vi "Swap DDS with CS.vi"(6 "Variant in":variant, 7 "Shift Pressed?":bool, 8 "error in (no error)":errorcluster, 10 "QD Combo Box Ref":refnum<vi>, 11 "QD Launch VI Ref":refnum<vi>) -> (0 "error out":errorcluster, 4 "Variant out":variant)   [LabVIEW 2017]
doc: "PLUGIN_DESCRIPTION: Replaces selected Diagram Disable Structure with Case Structure. Based on SAPHIR_DisableCode.vi from https://forums.ni.com/t5/SAPHIR-Toolkits-Documents/ViBox-Quick-Drop-datasheet/ta-p/3507939?profile.language=en\nPLUGIN_DEFAULT_SHORTCUT:"
uses:
  <userlib>/_LAVACR/Scripting Tools/Scripting Tools.lvlib
panel:
  in  "Undo Name":string="DisableCode"
  # "Created by https://github.com/Zieleslaw/, based on:"
  # "More informations on : https://decibel.ni.com/content/groups/saphir-toolkit"
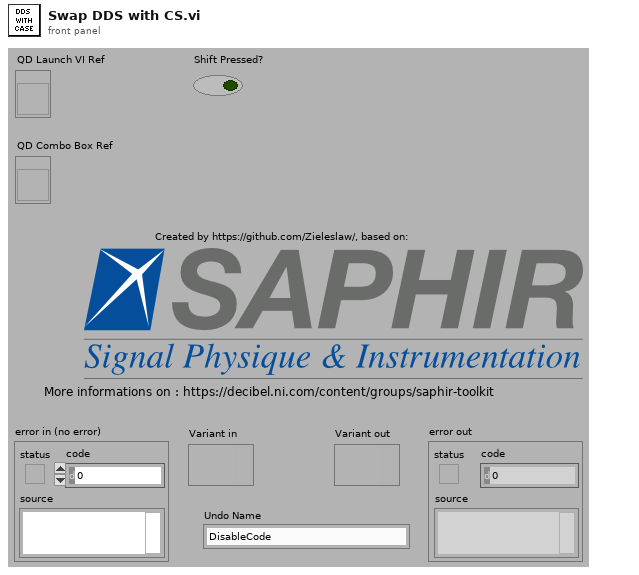
[diagram p1: front panel]
types:
  T1 = enum16{"Case Structure", "Stacked Sequence", "Event Structure", "Diagram Disable", "Conditional Disable", "While Loop", "For Loop", "Inplace Structure"}
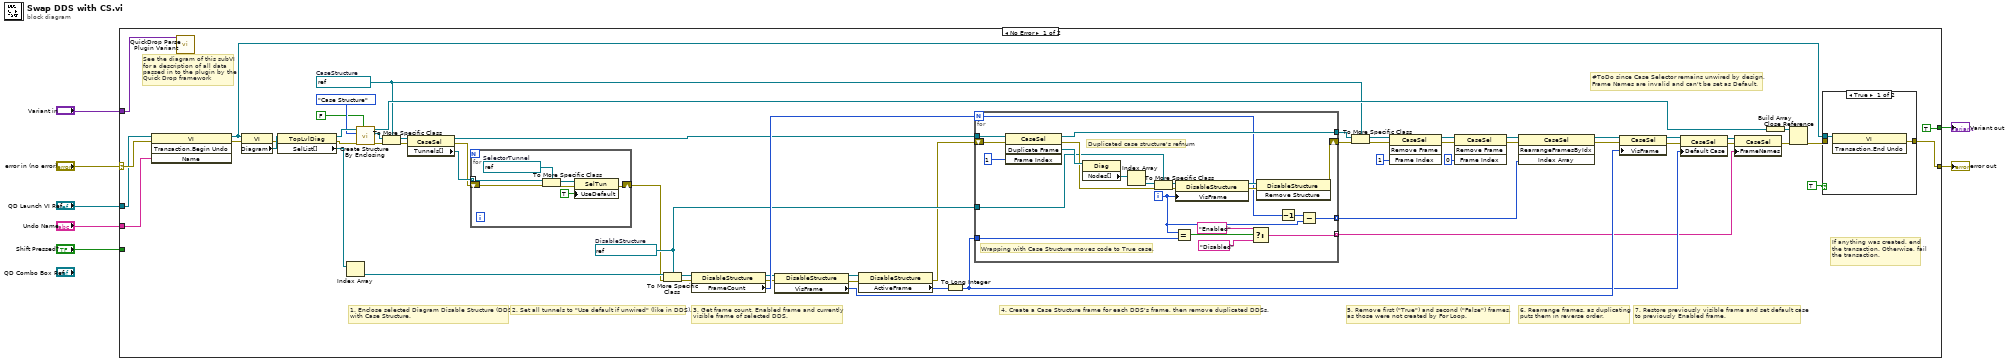
[diagram p0: block diagram]
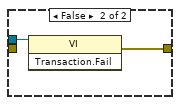
[diagram p2: hidden frame]
diagram:
  n1 = case shown="No Error" "error in (no error)" {
    selector: "error in (no error)" -> [w58 w102]
    tunnel: [w55 w102] -> w6
    tunnel: "QD Launch VI Ref" -> [w57 _]
    tunnel: "Variant in" -> [w59 _]
    tunnel: "Undo Name" -> [w56 _]
    tunnel: [TRUE _] -> w2
    tunnel: "Shift Pressed?" -> [_ _]
    frame No Error {
      w32 = refnum<vi> refnum  # DisableStructure
      w33 = refnum<vi> refnum  # CaseStructure
      # "2. Set all tunnels to \"Use default if unwired\" (like in DDS)."
      # "#ToDo since Case Selector remains unwired by design, \nFrame Names are invalid and can't be set as Default."
      # "6. Rearrange frames, as duplicating \nputs them in reverse order."
      # "5. Remove first (\"True\") and second (\"False\") frames, \nas those were not created by For Loop."
      # "7. Restore previously visible frame and set default case\nto previously Enabled frame."
      # "4. Create a Case Structure frame for each DDS's frame, then remove duplicated DDSs."
      # "3. Get frame count, Enabled frame and currently \nvisible frame of selected DDS."
      # "1. Enclose selected Diagram Disable Structure (DDS)\nwith Case Structure."
      # "If anything was created, end the transaction. Otherwise, fail the transaction."
      # "See the diagram of this subVI for a description of all data passed in to the plugin by the Quick Drop framework"
      n2 = invoke class="VI" method="Transaction.Begin Undo"(reference=w57, error in=w58, "Name"=w56) -> (reference out=w63:refnum<vi>, error out=w66:errorcluster)  [unwired: 1 in, 2 out]
      n3 = call <vilib>:"QuickDrop Parse Plugin Variant.vi"("QDKS Variant in"=w59) -> ()  [unwired: 12 in, 3 out]
      n4 = property class="VI"(reference=w63, error in=w66) -> (error out=w60:errorcluster, "Diagram"=w61:refnum<vi>)  [unwired: 1 out]
      n5 = property class="TopLvlDiag"(reference=w61, error in=w60) -> (reference out=w62:refnum<vi>, error out=w65:errorcluster, "SelList[]"=w53:refnum<vi>[])
      n6 = Index Array(array=w53) -> (element=w38:refnum<vi>)  [unwired: 1 in]
      n7 = call <userlib>:"Create Structure By Enclosing.vi"("Select everything except terminals ?"=FALSE, "error in (no error)"=w65, "Structure Type"=T1."Case Structure", "Diagram In"=w62) -> ("error out"=w49:errorcluster, "Structure Out"=w50:refnum<vi>, "Diagram Out"=w39:refnum<vi>)  [unwired: 5 in]
      n8 = To More Specific Class(target class=w33, reference=w50, error in=w49) -> (specific class reference=w12:refnum<vi>, error out=w44:errorcluster)
      n9 = property class="CaseSel"(reference=w12, error in=w44) -> (reference out=w11:refnum<vi>, error out=w9:errorcluster, "Tunnels[]"=w10:refnum<vi>[])
      n10 = for {
        tunnel: w10 -> [w68] mode=indexing
        shift-right: [w73] -> w8
        shift-left: w9 -> [w69]
        w74 = refnum<vi> refnum  # SelectorTunnel
        n11 = To More Specific Class(target class=w74, reference=w68, error in=w69) -> (specific class reference=w72:refnum<vi>, error out=w71:errorcluster)
        n12 = property class="SelTun"(reference=w72, error in=w71, "UseDefault"=TRUE ("Use Default if Unwired")) -> (error out=w73:errorcluster)  [unwired: 1 out]
      }
      n13 = To More Specific Class(target class=w32, reference=w38, error in=w8) -> (specific class reference=w47:refnum<vi>, error out=w45:errorcluster)
      n14 = property class="DisableStructure"(reference=w47, error in=w45) -> (reference out=w27:refnum<vi>, error out=w26:errorcluster, "FrameCount"=w46:i32)
      n15 = property class="DisableStructure"(reference=w27, error in=w26) -> (reference out=w21:refnum<vi>, error out=w40:errorcluster, "VisFrame"=w41:u32)
      n16 = property class="DisableStructure"(reference=w21, error in=w40) -> (error out=w22:errorcluster, "ActiveFrame"=w20:i16)  [unwired: 1 out]
      n17 = To Long Integer(number=w20) -> (32bit integer=w16:i32)
      n18 = for {
        N: w46 -> [w82]
        tunnel: [w87] -> w43
        tunnel: w11 -> [w97]
        shift-right: [w88] -> w42
        shift-left: w22 -> [w96]
        tunnel: w32 -> [w84]
        tunnel: [w81] -> w30 mode=indexing
        tunnel: w16 -> [w79]
        tunnel: [w75] -> w13 mode=indexing
        i -> [w80]
        # "Wrapping with Case Structure moves code to True case."
        # "Duplicated case structure's refnum"
        n19 = invoke class="CaseSel" method="Duplicate Frame"(reference=w97, error in=w96, "Frame Index"=u32 1) -> (reference out=w87:refnum<vi>, error out=w86:errorcluster, "Duplicate Frame"=w95:refnum<vi>)  [unwired: 1 in, 1 out]
        n20 = property class="Diag"(reference=w95) -> ("Nodes[]"=w94:refnum<vi>[])  [unwired: 1 in, 2 out]
        n21 = Index Array(array=w94) -> (element=w93:refnum<vi>)  [unwired: 1 in]
        n22 = To More Specific Class(target class=w84, reference=w93, error in=w86) -> (specific class reference=w92:refnum<vi>, error out=w91:errorcluster)
        n23 = property class="DisableStructure"(reference=w92, error in=w91, "VisFrame"=w80) -> (reference out=w90:refnum<vi>, error out=w89:errorcluster)
        n24 = Equal?(x=w80, y=w79) -> (x = y?=w78:bool)
        n25 = Select(t="Enabled", s=w78, f="Disabled") -> (s? t:f=w75:string)
        n26 = invoke class="DisableStructure" method="Remove Structure"(reference=w90, error in=w89) -> (error out=w88:errorcluster)  [unwired: 1 in, 2 out]
        n27 = Decrement(x=w82) -> (x-1=w83:i32)
        n28 = Subtract(x=w83, y=w80) -> (x-y=w81:i32)
      }
      n29 = To More Specific Class(target class=w33, reference=w43, error in=w42) -> (specific class reference=w25:refnum<vi>, error out=w24:errorcluster)
      n30 = invoke class="CaseSel" method="Remove Frame"(reference=w25, error in=w24, "Frame Index"=u32 1) -> (reference out=w35:refnum<vi>, error out=w37:errorcluster)  [unwired: 1 in, 2 out]
      n31 = invoke class="CaseSel" method="Remove Frame"(reference=w35, error in=w37, "Frame Index"=u32 0) -> (reference out=w31:refnum<vi>, error out=w36:errorcluster)  [unwired: 1 in, 2 out]
      n32 = invoke class="CaseSel" method="RearrangeFramesByIdx"(reference=w31, error in=w36, "Index Array"=w30) -> (reference out=w29:refnum<vi>, error out=w28:errorcluster)  [unwired: 1 in, 2 out]
      n33 = property class="CaseSel"(reference=w29, error in=w28, "VisFrame"=w41) -> (reference out=w18:refnum<vi>, error out=w19:errorcluster)
      n34 = property class="CaseSel"(reference=w18, error in=w19, "Default Case"=w16) -> (reference out=w14:refnum<vi>, error out=w17:errorcluster)
      n35 = property class="CaseSel"(reference=w14, error in=w17, "FrameNames"=w13) -> (error out=w15:errorcluster)  [unwired: 1 out]
      n36 = Build Array(w39) -> (w48:refnum<vi>[])
      n37 = Close Reference(reference=w48, error in (no error)=w15) -> (error out=w64:errorcluster)
      n38 = case shown="True" TRUE ("x") {
        tunnel: w63 -> [w98 w100]
        tunnel: [w99 w101] -> w55
        tunnel: w64 -> [_ _]
        frame True {
          n39 = invoke class="VI" method="Transaction.End Undo"(reference=w98) -> (error out=w99:errorcluster)  [unwired: 2 in, 2 out]
        }
        frame False {
          n40 = invoke class="VI" method="Transaction.Fail"(reference=w100) -> (error out=w101:errorcluster)  [unwired: 2 in, 2 out]
        }
      }
    }
    frame Error {
    }
  }
  "error out" <- w6
  "Variant out" <- w2
